vi "Act 4.vi"() -> ()   [LabVIEW 2010]
panel:
  out "Deg F":dbl
  in  "Deg C":dbl
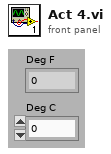
[diagram p1: front panel]
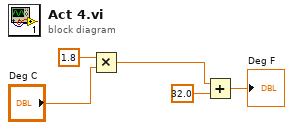
[diagram p0: block diagram]
diagram:
  n1 = Multiply(x=1.8, y="Deg C") -> (x*y=w3:dbl)
  n2 = Add(x=w3, y=32.0) -> (x+y=→"Deg F":dbl)
